vi "Asset Test.vi"() -> ()   [LabVIEW 2019]
panel:
  out "clos":u32
  out "init":u32
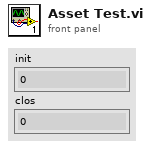
[diagram p1: front panel]
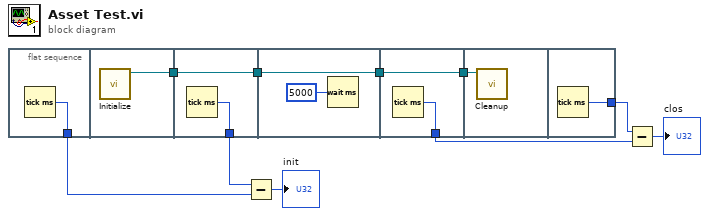
[diagram p0: block diagram]
diagram:
  n1 = flat-sequence {
    tunnel: [w11] -> w8
    tunnel: [w12] -> w6
    tunnel: w6 -> [w14]
    tunnel: [w14] -> w5
    tunnel: [w13] -> w4
    tunnel: w5 -> [w16]
    tunnel: [w16] -> w3
    tunnel: w3 -> [w18]
    tunnel: [w18] -> w2
    tunnel: [w17] -> w1
    tunnel: w2 -> [w19]
    tunnel: [w20] -> w7
    frame #0 {
      n2 = Tick Count (ms)() -> (millisecond timer value=w11:u32)
    }
    frame #1 {
      n3 = call "Initialize.vi"() -> ("asset utilization"=w12:refnum<class "NI SystemLink Asset Utilization.lvclass">)  [unwired: 11 in]
    }
    frame #2 {
      n4 = Tick Count (ms)() -> (millisecond timer value=w13:u32)
    }
    frame #3 {
      n5 = Wait (ms)(milliseconds to wait=u32 5000) -> ()  [unwired: 1 out]
    }
    frame #4 {
      n6 = Tick Count (ms)() -> (millisecond timer value=w17:u32)
    }
    frame #5 {
      n7 = call "Cleanup.vi"("asset utilization"=w19) -> ()  [unwired: 11 in]
    }
    frame #6 {
      n8 = Tick Count (ms)() -> (millisecond timer value=w20:u32)
    }
  }
  n9 = Subtract(x=w4, y=w8) -> (x-y=→"init":u32)
  n10 = Subtract(x=w7, y=w1) -> (x-y=→"clos":u32)
